vi "UART Init.vi"(4 "TX GPIO":T1=16, 5 "Term Char (None)":string, 6 "RX GPIO":T1=17, 7 "UART #":T2, 8 "error in (no error)":errorcluster, 10 "Baud":u32=115200, 11 "VisaComms in":refnum<class "VisaComms.lvclass">) -> (0 "error out":errorcluster, 3 "VisaComms out":refnum<class "VisaComms.lvclass">)   [LabVIEW 2020, in "CTI.lvlib" / "VisaComms.lvclass"]
uses:
  VisaComms.lvclass
  UART Number.ctl
  GPIO Number.ctl
  VisaComms.lvclass/VisaComms.ctl
  CTI.lvlib
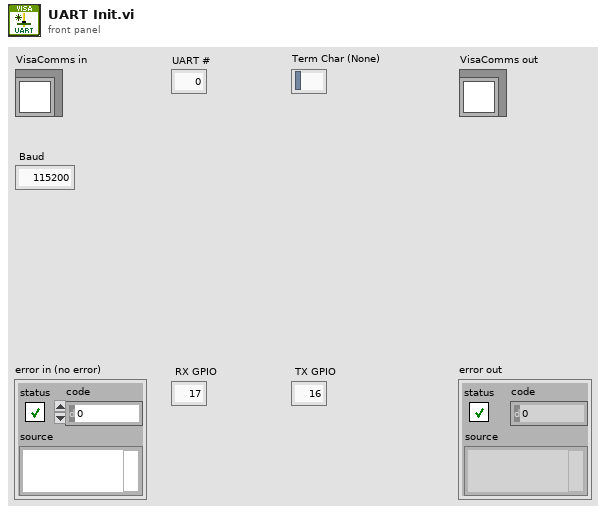
[diagram p1: front panel]
types:
  T1 = typedef "CTI.lvlib/GPIO Number.ctl" = i8
  T2 = typedef "CTI.lvlib/UART Number.ctl" = i8
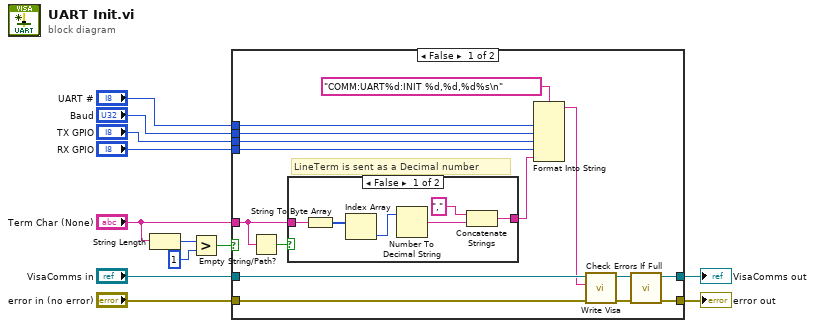
[diagram p0: block diagram]
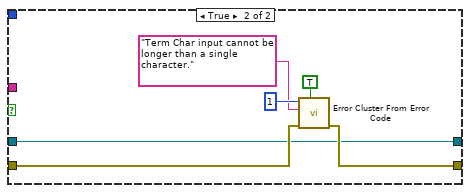
[diagram p3: hidden frame]
diagram:
  n1 = String Length(string="Term Char (None)") -> (length=w12:i32)
  n2 = Greater?(x=w12, y=1) -> (0:w10:bool)
  n3 = case shown="False" w10 {
    tunnel: "UART #" -> [w26 _]
    tunnel: "Baud" -> [w25 _]
    tunnel: "TX GPIO" -> [w24 _]
    tunnel: "RX GPIO" -> [w23 _]
    tunnel: "Term Char (None)" -> [w21 _]
    tunnel: "error in (no error)" -> [w20 w39]
    tunnel: [w15 w38] -> w6
    tunnel: "VisaComms in" -> [w17 w34]
    tunnel: [w13 w34] -> w7
    frame False {
      # "LineTerm is sent as a Decimal number"
      n4 = Empty String/Path?(string/path=w21) -> (empty?=w22:bool)
      n5 = case shown="False" w22 {
        tunnel: w21 -> [w31 _]
        tunnel: [w33 _] -> w18
        frame False {
          n6 = String To Byte Array(string=w31) -> (unsigned byte array=w30:u8[])
          n7 = Index Array(array=w30) -> (element=w29:u8)  [unwired: 1 in]
          n8 = Number To Decimal String(number=w29) -> (decimal integer string=w28:string)  [unwired: 1 in]
          n9 = Concatenate Strings("," ("string"), w28) -> (w33:string)
        }
        frame True {
        }
      }
      n10 = Format Into String(format string="COMM:UART%d:INIT %d,%d,%d%s\n", w26, w25, w24, w23, w18) -> (resulting string=w16:string)  [unwired: 2 in, 1 out]
      n11 = call "Write Visa.vi"("error in (no error)"=w20, "write buffer"=w16, "VisaComms in"=w17) -> ("error out"=w19:errorcluster, "VisaComms out"=w14:refnum<class "VisaComms.lvclass">)  [unwired: 6 in, 1 out]
      n12 = call "Check Errors If Full.vi"("error in (no error)"=w19, "VisaComms in"=w14) -> ("error out"=w15:errorcluster, "VisaComms out"=w13:refnum<class "VisaComms.lvclass">)  [unwired: 8 in]
    }
    frame True {
      n13 = call <vilib>:"Error Cluster From Error Code.vi"("show call chain? (False)"=TRUE, "error in (no error)"=w39, "error message (\"\")"="Term Char input cannot be longer than a single character.", "error code (0)"=1) -> ("error out"=w38:errorcluster)  [unwired: 5 in]
    }
  }
  "error out" <- w6
  "VisaComms out" <- w7
